vi "Exit Library.vi"(8 "error in":errorcluster) -> (0 "error out":errorcluster, 3 "exit error code":i32)   [LabVIEW 2020, in "AIM ARINC 429 Hardware API.lvlib"]
uses:
  AIM ARINC 429 Hardware API.lvlib
  <instrlib>/AIM GmbH/ARINC-429/AIM429LV.lvlib
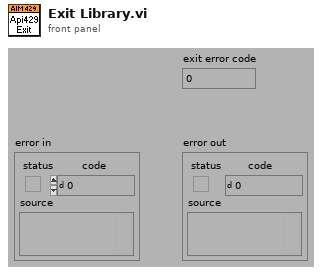
[diagram p1: front panel]
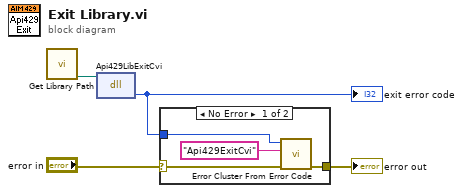
[diagram p0: block diagram]
diagram:
  n1 = call <instrlib>:"Get Library Path.vi"() -> ("GlobalDLLPath"=w1:path)  [unwired: 11 in]
  n2 = dll-call lib="api_civ.9.dll" fn="Api429LibExitCvi"(path in=w1) -> ("error code"=w2:i32)  [unwired: 2 in, 2 out]
  "exit error code" <- w2
  n3 = case shown="No Error" "error in" {
    selector: "error in" -> [w8 w9]
    tunnel: [w7 w9] -> w3
    tunnel: w2 -> [w5 _]
    frame No Error {
      n4 = call <vilib>:"Error Cluster From Error Code.vi"("error in (no error)"=w8, "error message (\"\")"="Api429ExitCvi", "error code (0)"=w5) -> ("error out"=w7:errorcluster)  [unwired: 6 in]
    }
    frame Error {
    }
  }
  "error out" <- w3
